vi "Set gRPC ID.vi"(10 "gRPC ID":T1, 11 "gRPC server in":refnum<class "Servicer.lvclass">) -> (3 "gRPC server out":refnum<class "Servicer.lvclass">)   [LabVIEW 2019, in "gRPC-servicer.lvlib" / "Servicer.lvclass"]
uses:
  Servicer.lvclass
  gRPC lv Support/Shared/grpcId.ctl
  Servicer.lvclass/Servicer.ctl
  gRPC lv Support/grpc-lvsupport.lvlib
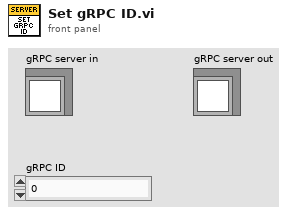
[diagram p1: front panel]
types:
  T1 = typedef "grpc-lvsupport.lvlib/grpcId.ctl" = u64
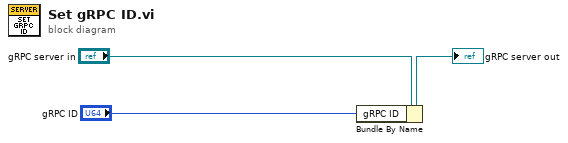
[diagram p0: block diagram]
diagram:
  n1 = Bundle By Name(cluster="gRPC server in", "gRPC ID"="gRPC ID") -> (→"gRPC server out":refnum<class "Servicer.lvclass">)
